vi "CMN_ReadGblsFromFile.vi"(8 "error in (no error)":errorcluster, 10 "database name":string="DBS", 11 "configuration file path":path=path "/home/ArcVIEW/ConfigFiles/ctiocameragui.cfg") -> (0 "error out":errorcluster)   [LabVIEW 2016]
uses:
  <vilib>/Utility/config.llb/Read Key (String).vi
  DBSHAND/private/vis/DatabaseHand_Element_Set(string).vi
  <vilib>/Utility/config.llb/NI_LVConfig.lvlib
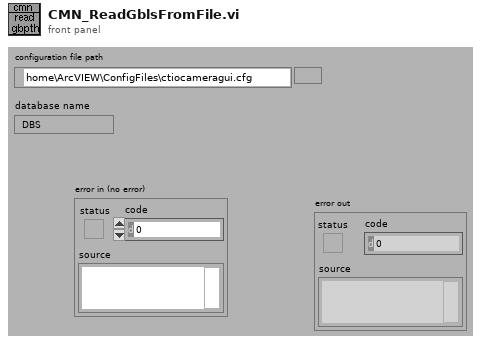
[diagram p1: front panel]
types:
  T1 = typedef "NI_LVConfig.lvlib/Config Data RefNum.ctl" = refnum<k1>
  T2 = typedef "DatabaseHand_RefNum.ctl" = refnum<vi>
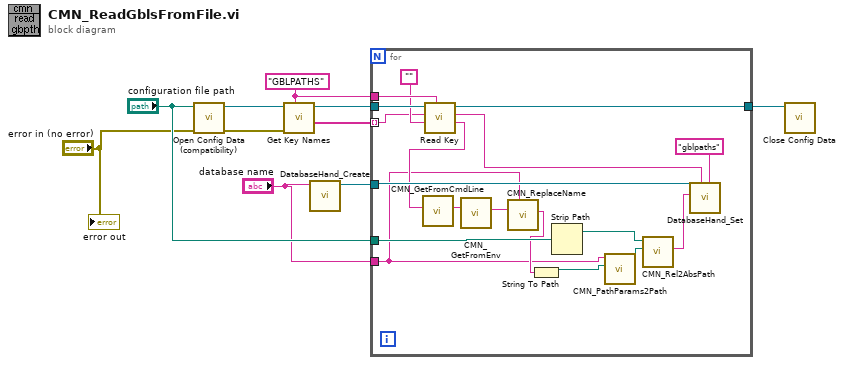
[diagram p0: block diagram]
diagram:
  w6 = "GBLPATHS" ("section")
  n1 = call <vilib>:"Open Config Data (compatibility).vi"("error in (no error)"="error in (no error)", "configuration file path"="configuration file path") -> ("error out"=w9:errorcluster, "refnum"=w10:T1)  [unwired: 7 in, 1 out]
  n2 = call <vilib>:"Get Key Names.vi"("section"=w6, "error in (no error)"=w9, "refnum"=w10) -> ("key names"=w8:string[], "refnum out"=w7:T1)  [unwired: 7 out]
  n3 = call "DatabaseHand_Create.vi"("Name"="database name") -> ("Database RefNum out"=w5:T2)  [unwired: 1 in, 9 out]
  n4 = for {
    tunnel: w8 -> [w22] mode=indexing
    tunnel: w7 -> [w27]
    tunnel: w6 -> [w26]
    tunnel: w5 -> [w24]
    tunnel: "configuration file path" -> [w18]
    tunnel: "database name" -> [w11]
    tunnel: [w16] -> w2
    n5 = call-poly <vilib>:"Read Key.vi"("section"=w26, "default value"="", "key"=w22, "refnum"=w27) -> ("value"=w14:string, "refnum out"=w16:T1)  [unwired: 2 in, 4 out]
    n6 = call "CMN_GetFromCmdLine.vi"("str in"=w14) -> ("str out"=w15:string)  [unwired: 10 out]
    n7 = call "CMN_GetFromEnv.vi"("str in"=w15) -> ("str out"=w13:string)  [unwired: 10 out]
    n8 = call "CMN_ReplaceName.vi"("DBS"=w11, "name in"=w13) -> ("name out"=w12:string)  [unwired: 9 out]
    n9 = String To Path(string=w12) -> (path=w20:path)
    n10 = Strip Path(path=w18) -> (stripped path=w19:path)  [unwired: 1 out]
    n11 = call "CMN_PathParams2Path.vi"("Path In"=w20, "Dabatase name"=w11) -> ("Path out"=w21:path)  [unwired: 1 in, 8 out]
    n12 = call "CMN_Rel2AbsPath.vi"("test path"=w21, "absolute path"=w19) -> ("output path (str)"=w17:string)  [unwired: 1 in, 8 out]
    n13 = call-poly "DatabaseHand_Set.vi"("group"="gblpaths", "name"=w22, "value"=w17, "Database RefNum in"=w24) -> ()  [unwired: 4 in, 4 out]
  }
  n14 = call <vilib>:"Close Config Data.vi"("refnum"=w2) -> ()  [unwired: 2 in, 9 out]
  "error out" <- "error in (no error)"
